vi "BinAvgSub3.vi"(7 "Extend to 0":bool, 9 "Bin size":dbl, 10 "X coumn index":i32, 11 "Data in":dbl[][](array[numeric])) -> (3 "Binned data":dbl[][](array[numeric]) format="%#_10g")   [LabVIEW 2018]
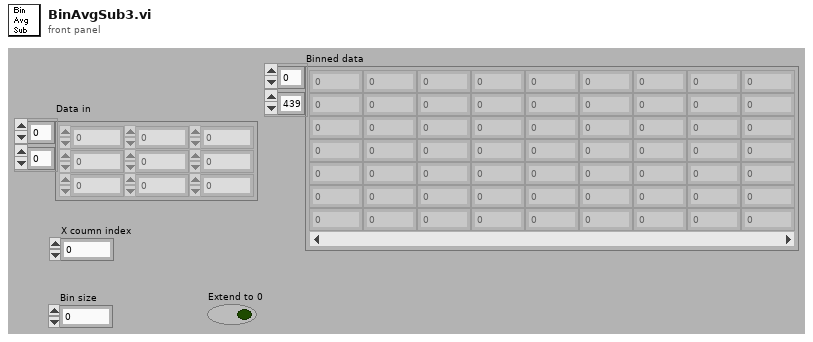
[diagram p1: front panel]
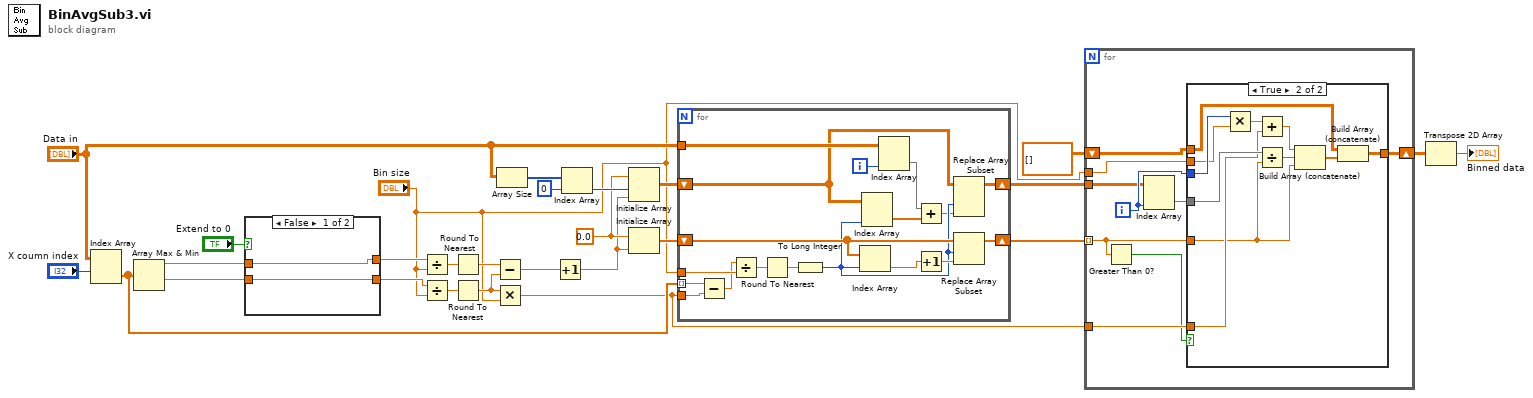
[diagram p0: block diagram]
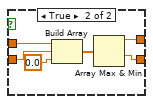
[diagram p3: hidden frame]
diagram:
  w13 = 0.0 ("element")
  n1 = Index Array(array="Data in", index (row)="X coumn index") -> (element=w16:dbl[])  [unwired: 1 in]
  n2 = Array Max & Min(array=w16) -> (max value=w23:dbl, min value=w22:dbl)  [unwired: 2 out]
  n3 = case shown="False" "Extend to 0" {
    tunnel: w23 -> [w29 w35]
    tunnel: w22 -> [w28 w34]
    tunnel: [w29 w31] -> w20
    tunnel: [w28 w30] -> w21
    frame False {
    }
    frame True {
      n4 = Build Array(w35, w34, 0.0 ("element")) -> (w32:dbl[])
      n5 = Array Max & Min(array=w32) -> (max value=w31:dbl, min value=w30:dbl)  [unwired: 2 out]
    }
  }
  n6 = Divide(x=w20, y="Bin size") -> (x/y=w19:dbl)
  n7 = Divide(x=w21, y="Bin size") -> (x/y=w18:dbl)
  n8 = Round To Nearest(number=w19) -> (nearest integer value=w17:dbl)
  n9 = Round To Nearest(number=w18) -> (nearest integer value=w10:dbl)
  n10 = Subtract(x=w17, y=w10) -> (x-y=w12:dbl)
  n11 = Multiply(x=w10, y="Bin size") -> (x*y=w7:dbl)
  n12 = Array Size(array="Data in") -> (size(s)=w26:i32[])
  n13 = Increment(x=w12) -> (x+1=w5:dbl)
  n14 = Index Array(array=w26, index=0) -> (element=w14:i32)
  n15 = Initialize Array(w13, w14, w5) -> (w15:dbl[][])
  n16 = Initialize Array(w13, w5) -> (w11:dbl[])
  n17 = for {
    tunnel: w16 -> [w38] mode=indexing
    shift-right: [w46] -> w4
    shift-left: w15 -> [w47]
    tunnel: "Data in" -> [w53]
    tunnel: "Bin size" -> [w51]
    tunnel: w7 -> [w37]
    shift-right: [w45] -> w9
    shift-left: w11 -> [w44]
    i -> [w52]
    n18 = Subtract(x=w38, y=w37) -> (x-y=w39:dbl)
    n19 = Divide(x=w39, y=w51) -> (x/y=w50:dbl)
    n20 = Round To Nearest(number=w50) -> (nearest integer value=w36:dbl)
    n21 = To Long Integer(number=w36) -> (32bit integer=w42:i32)
    n22 = Index Array(array=w44, index=w42) -> (element=w48:dbl)
    n23 = Index Array(array=w47, index (col)=w42) -> (element=w41:dbl[])  [unwired: 1 in]
    n24 = Index Array(array=w53, index (col)=w52) -> (element=w49:dbl[])  [unwired: 1 in]
    n25 = Add(x=w49, y=w41) -> (x+y=w40:dbl[])
    n26 = Increment(x=w48) -> (x+1=w43:dbl)
    n27 = Replace Array Subset(array=w47, new element=w40, index (col)=w42) -> (w46:dbl[][])  [unwired: 1 in]
    n28 = Replace Array Subset(array=w44, new element=w43, index=w42) -> (w45:dbl[])
  }
  n29 = for {
    tunnel: w9 -> [w54] mode=indexing
    tunnel: "Bin size" -> [w60]
    tunnel: w7 -> [w59]
    shift-right: [w57] -> w2
    shift-left: dbl[][] [] -> [w56]
    tunnel: w4 -> [w58]
    i -> [w61]
    n30 = Greater Than 0?(x=w54) -> (x > 0?=w55:bool)
    n31 = Index Array(array=w58, index (col)=w61) -> (element=w62:dbl[])  [unwired: 1 in]
    n32 = case shown="True" w55 {
      tunnel: w62 -> [_ w74]
      tunnel: w61 -> [_ w73]
      tunnel: w60 -> [_ w72]
      tunnel: w59 -> [_ w71]
      tunnel: w54 -> [_ w67]
      tunnel: [w63 w66] -> w57
      tunnel: w56 -> [w63 w64]
      frame False {
      }
      frame True {
        n33 = Multiply(x=w73, y=w72) -> (x*y=w70:dbl)
        n34 = Add(x=w70, y=w71) -> (x+y=w69:dbl)
        n35 = Divide(x=w74, y=w67) -> (x/y=w68:dbl[])
        n36 = Build Array (concatenate)(w69, w68, w67) -> (w65:dbl[])
        n37 = Build Array (concatenate)(w64, w65) -> (w66:dbl[][])
      }
    }
  }
  n38 = Transpose 2D Array(2D array=w2) -> (transposed array=→"Binned data":dbl[][])
